vi "seterrors.vi"(0 "error IO":errorcluster) -> ()   [LabVIEW 2015]
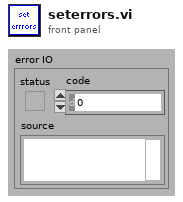
[diagram p1: front panel]
types:
  T1 = cluster{"AO":refnum<k21>[], "E_AO":errorcluster[]}
  T2 = cluster{" AI":refnum<k21>, "E_AI":errorcluster, "header":dbl[]}
  T3 = cluster{"upleft":bool, "up":bool, "upright":bool, "right":bool, "downright":bool, "down":bool, "downleft":bool, "left":bool, "Bigsmall":bool, "E_stage":errorcluster}
  T4 = cluster{"CI":refnum<k21>[], "E_CI":errorcluster[]}
  T5 = cluster{"filetif":refnum<file>[], "E_filetif":errorcluster[]}
  T6 = cluster{"E_binfile":errorcluster[], "binfile":refnum<file>[]}
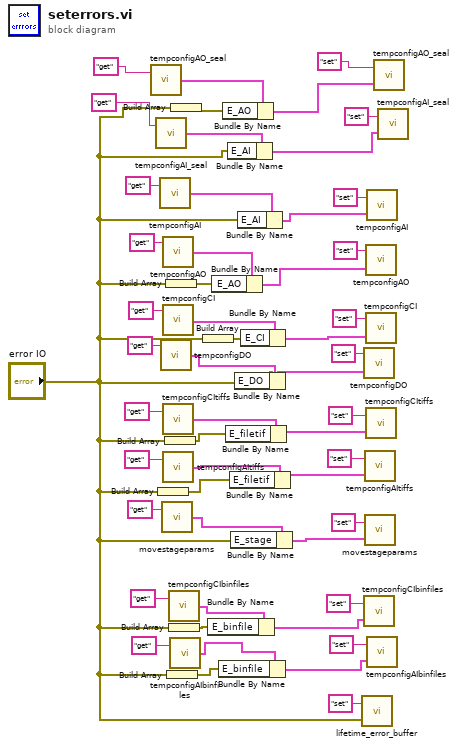
[diagram p0: block diagram]
diagram:
  n1 = call "tempconfigAO_seal.vi"("command"="get") -> ("Temp Config out"=w8:T1)  [unwired: 1 in]
  n2 = call "tempconfigAI_seal.vi"("command"="get") -> ("Temp Config out"=w7:T2)  [unwired: 1 in]
  n3 = Build Array("error IO") -> (w22:errorcluster[])
  n4 = call "tempconfigAI.vi"("command"="get") -> ("Temp Config out"=w48:T2)  [unwired: 1 in]
  n5 = call "tempconfigDO.vi"("command"="get") -> ("Temp Config out"=w45:cluster{"DO":refnum<k21>, "E_DO":errorcluster})  [unwired: 1 in]
  n6 = call "movestageparams.vi"("command"="get") -> ("Params out"=w44:T3)  [unwired: 1 in]
  n7 = call "tempconfigAO.vi"("command"="get") -> ("Temp Config out"=w47:T1)  [unwired: 1 in]
  n8 = call "tempconfigCI.vi"("command"="get") -> ("Temp Config out"=w46:T4)  [unwired: 1 in]
  n9 = call "tempconfigCItiffs.vi"("command"="get") -> ("Temp Config out"=w29:T5)  [unwired: 1 in]
  n10 = call "tempconfigAItiffs.vi"("command"="get") -> ("Temp Config out"=w28:T5)  [unwired: 1 in]
  n11 = Build Array("error IO") -> (w23:errorcluster[])
  n12 = Build Array("error IO") -> (w11:errorcluster[])
  n13 = Build Array("error IO") -> (w14:errorcluster[])
  n14 = call "tempconfigCIbinfiles.vi"("command"="get") -> ("Temp Config out"=w17:T6)  [unwired: 1 in]
  n15 = Build Array("error IO") -> (w15:errorcluster[])
  n16 = call "tempconfigAIbinfiles.vi"("command"="get") -> ("Temp Config out"=w16:T6)  [unwired: 1 in]
  n17 = Build Array("error IO") -> (w6:errorcluster[])
  n18 = Build Array("error IO") -> (w32:errorcluster[])
  n19 = Bundle By Name(cluster=w17, "E_binfile"=w15) -> (w13:T6)
  n20 = Bundle By Name(cluster=w47, "E_AO"=w11) -> (w37:T1)
  n21 = Bundle By Name(cluster=w16, "E_binfile"=w14) -> (w12:T6)
  n22 = Bundle By Name(cluster=w8, "E_AO"=w6) -> (w1:T1)
  n23 = Bundle By Name(cluster=w29, "E_filetif"=w23) -> (w24:T5)
  n24 = Bundle By Name(cluster=w7, "E_AI"="error IO") -> (w2:T2)
  n25 = Bundle By Name(cluster=w28, "E_filetif"=w22) -> (w25:T5)
  n26 = Bundle By Name(cluster=w44, "E_stage"="error IO") -> (w34:T3)
  n27 = Bundle By Name(cluster=w45, "E_DO"="error IO") -> (w35:cluster{"DO":refnum<k21>, "E_DO":errorcluster})
  n28 = Bundle By Name(cluster=w48, "E_AI"="error IO") -> (w38:T2)
  n29 = Bundle By Name(cluster=w46, "E_CI"=w32) -> (w36:T4)
  n30 = call "lifetime_error_buffer.vi"("error in"="error IO", "command"="set") -> ()  [unwired: 1 out]
  n31 = call "tempconfigDO.vi"("Temp Config in"=w35, "command"="set") -> ()  [unwired: 1 out]
  n32 = call "tempconfigCIbinfiles.vi"("Temp Config in"=w13, "command"="set") -> ()  [unwired: 1 out]
  n33 = call "tempconfigAItiffs.vi"("Temp Config in"=w25, "command"="set") -> ()  [unwired: 1 out]
  n34 = call "movestageparams.vi"("Params in"=w34, "command"="set") -> ()  [unwired: 1 out]
  n35 = call "tempconfigAO.vi"("Temp Config in"=w37, "command"="set") -> ()  [unwired: 1 out]
  n36 = call "tempconfigCI.vi"("Temp Config in"=w36, "command"="set") -> ()  [unwired: 1 out]
  n37 = call "tempconfigCItiffs.vi"("Temp Config in"=w24, "command"="set") -> ()  [unwired: 1 out]
  n38 = call "tempconfigAI.vi"("Temp Config in"=w38, "command"="set") -> ()  [unwired: 1 out]
  n39 = call "tempconfigAIbinfiles.vi"("Temp Config in"=w12, "command"="set") -> ()  [unwired: 1 out]
  n40 = call "tempconfigAO_seal.vi"("Temp Config in"=w1, "command"="set") -> ()  [unwired: 1 out]
  n41 = call "tempconfigAI_seal.vi"("Temp Config in"=w2, "command"="set") -> ()  [unwired: 1 out]
